vi "onTestExecution.vi"(8 "error in (no error)":errorcluster, 11 "Unit Tests for Runner in":refnum<class "Unit Tests for Runner.lvclass">) -> (0 "error out":errorcluster, 3 "Unit Tests for Runner out":refnum<class "Unit Tests for Runner.lvclass">)   [LabVIEW 2013, in "Unit Tests for Runner.lvclass"]
uses:
  Unit Tests for Runner.lvclass
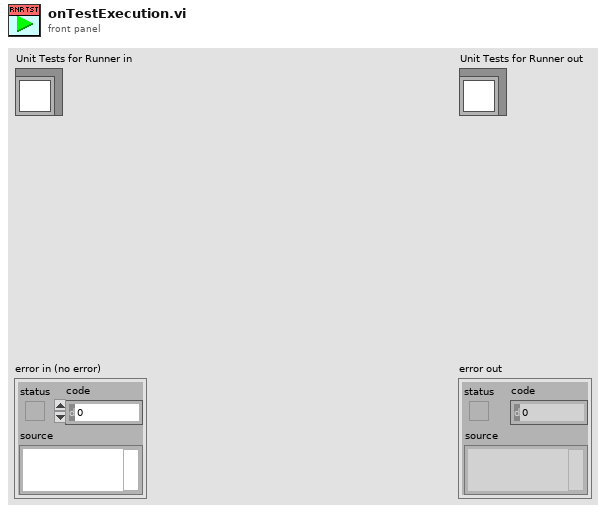
[diagram p1: front panel]
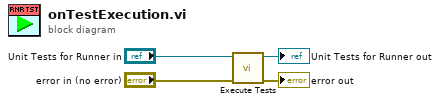
[diagram p0: block diagram]
diagram:
  n1 = call-dynamic "Execute Tests.vi"("error in (no error)"="error in (no error)", "Unit Tests for Runner in"="Unit Tests for Runner in") -> ("error out"=→"error out":errorcluster, "Unit Tests for Runner out"=→"Unit Tests for Runner out":refnum<class "Unit Tests for Runner.lvclass">)  [unwired: 8 in]
